vi "create output file.vi"(10 "session name\n(optional; no special characters)":string, 11 "input path":path) -> (3 "refnum out":refnum<file>)   [LabVIEW 2013]
panel:
  out "error out":errorcluster
  in  "error in":errorcluster
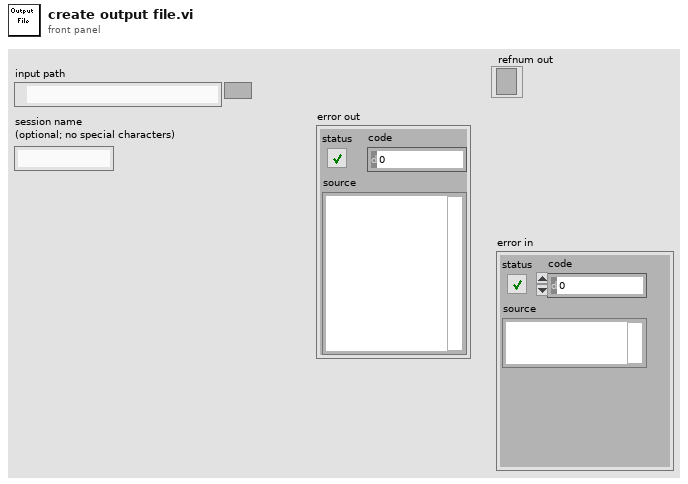
[diagram p1: front panel]
types:
  T1 = enum16{"open", "replace", "create", "open or create", "replace or create", "replace or create with confirmation"}
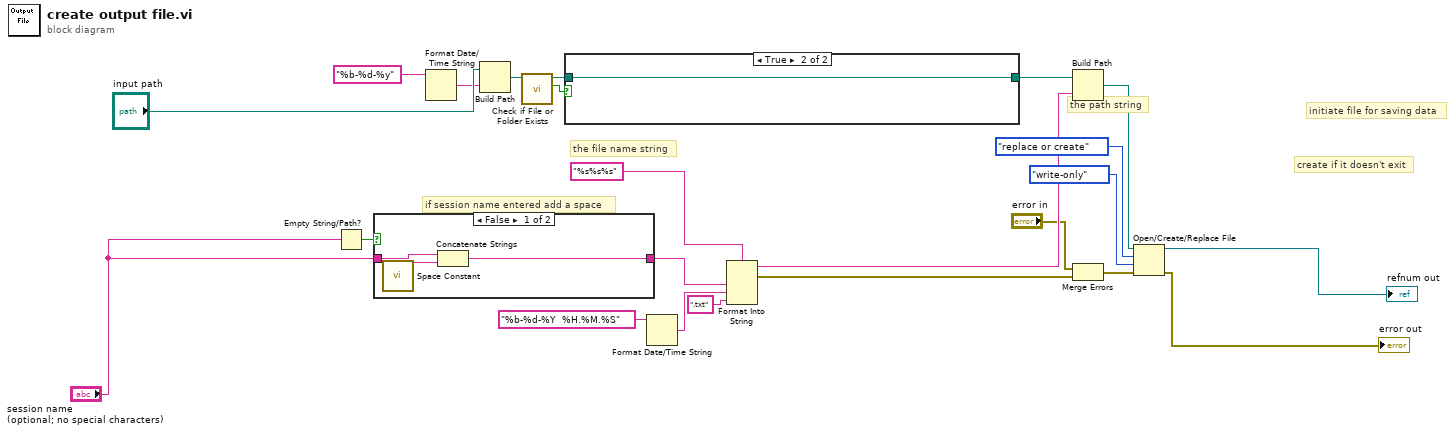
[diagram p0: block diagram]
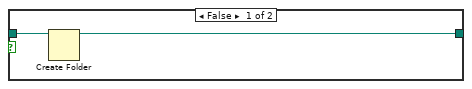
[diagram p3: hidden frame]
diagram:
  # "initiate file for saving data"
  # "if session name entered add a space"
  # "the path string"
  # "the file name string"
  # "create if it doesn't exit"
  n1 = Empty String/Path?(string/path="session name\n(optional; no special characters)") -> (empty?=w3:bool)
  n2 = case shown="False" w3 {
    tunnel: "session name\n(optional; no special characters)" -> [w26 w27]
    tunnel: [w25 w27] -> w1
    frame False {
      n3 = call <vilib>:"Space Constant.vi"() -> ("String"=w24:string)
      n4 = Concatenate Strings(w26, w24) -> (w25:string)
    }
    frame True {
    }
  }
  n5 = Format Date/Time String(time format string (%c)="%b-%d-%y") -> (date/time string=w7:string)  [unwired: 2 in]
  n6 = Build Path(base path="input path", name or relative path=w7) -> (appended path=w9:path)
  n7 = call <vilib>:"Check if File or Folder Exists.vi"("path"=w9) -> ("file or folder exists?"=w12:bool, "dup path"=w6:path)  [unwired: 8 in, 1 out]
  n8 = case shown="True" w12 {
    tunnel: w6 -> [w29 w30]
    tunnel: [w28 w30] -> w11
    frame False {
      n9 = Create Folder(path (use dialog)=w29) -> (created path=w28:path)  [unwired: 2 in, 2 out]
    }
    frame True {
    }
  }
  n10 = Format Date/Time String(time format string (%c)="%b-%d-%Y  %H.%M.%S") -> (date/time string=w4:string)  [unwired: 2 in]
  n11 = Format Into String(format string="%s%s%s", w1, w4, ".txt" ("input 2")) -> (resulting string=w21:string, error out=w20:errorcluster)  [unwired: 2 in]
  n12 = Build Path(base path=w11, name or relative path=w21) -> (appended path=w19:path)
  n13 = Merge Errors("error in", w20) -> (w14:errorcluster)
  n14 = Open/Create/Replace File(file path (use dialog)=w19, error in=w14, operation (0:open)=T1."replace or create", access (0:read/write)=enum16{"read/write", "read-only", "write-only"}."write-only") -> (refnum out=→"refnum out":refnum<file>, error out=→"error out":errorcluster)  [unwired: 2 in, 1 out]
